vi "test1_korras.vi"() -> ()   [LabVIEW 2012]
panel:
  out "XY Graph 2":cluster{timestamp[], dbl[]}(graph)
  out "XY Graph":cluster{timestamp[], dbl[]}(graph)
  in  "Path":path
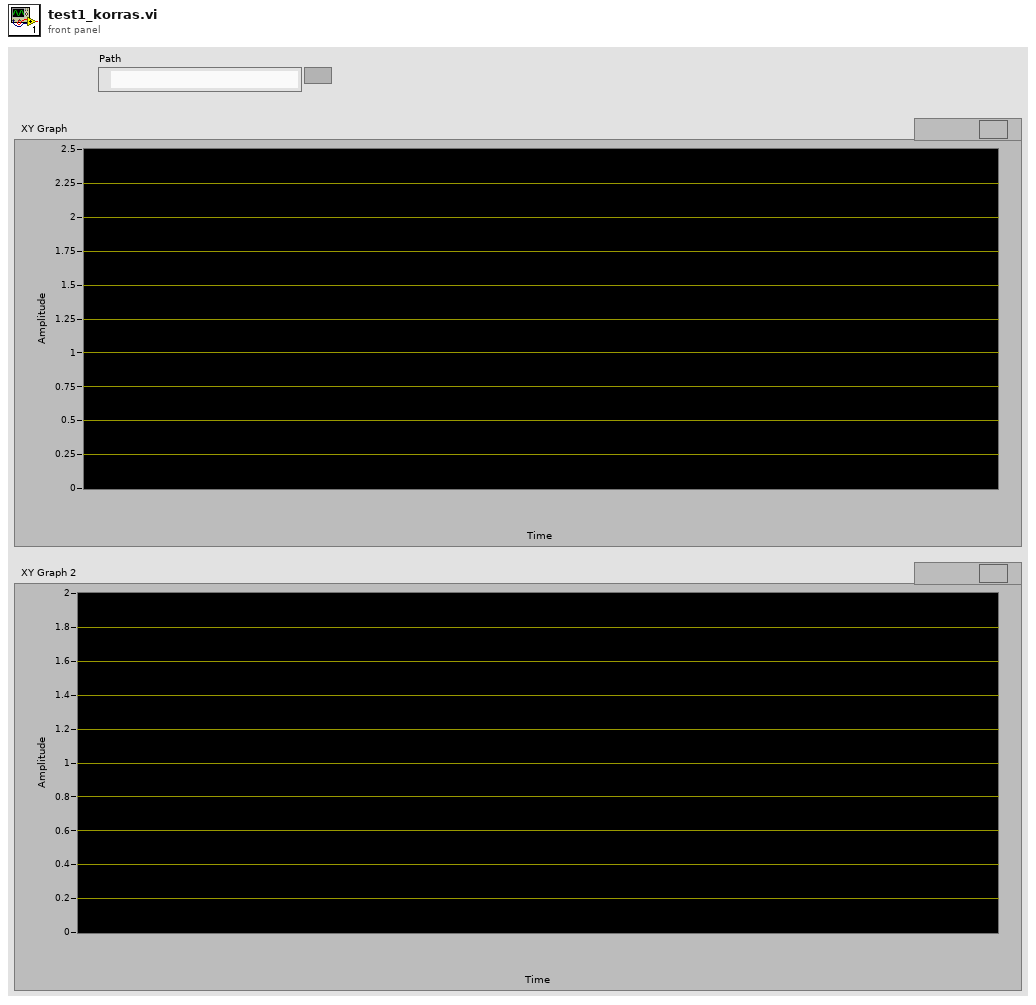
[diagram p1: front panel]
types:
  T1 = enum16{"open", "replace", "create", "open or create", "replace or create", "replace or create with confirmation"}
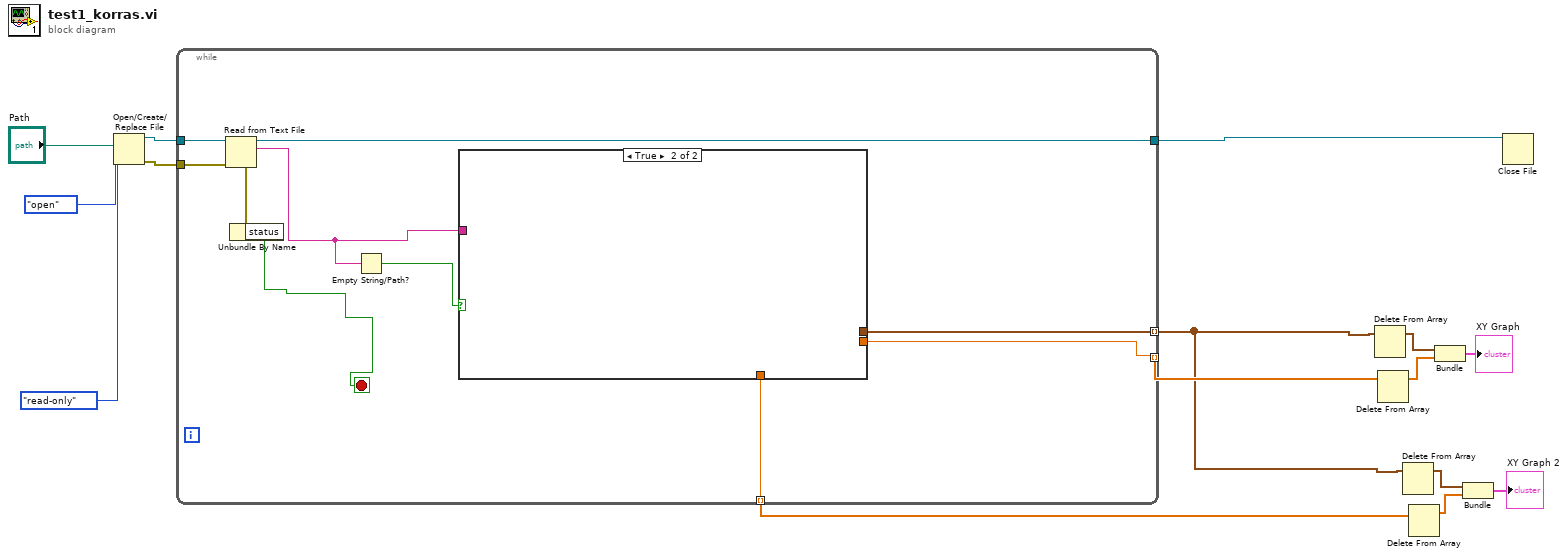
[diagram p0: block diagram]
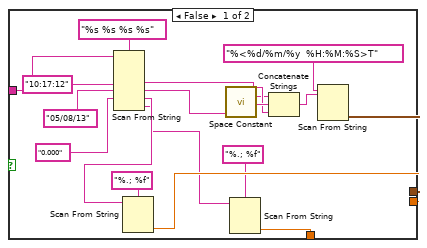
[diagram p2: hidden frame]
diagram:
  n1 = Open/Create/Replace File(file path (use dialog)="Path", operation (0:open)=T1."open", access (0:read/write)=enum16{"read/write", "read-only", "write-only"}."read-only") -> (refnum out=w14:refnum<file>, error out=w15:errorcluster)  [unwired: 3 in, 1 out]
  n2 = while {
    tunnel: w15 -> [w25]
    tunnel: w14 -> [w23]
    tunnel: [w22] -> w10
    tunnel: [w20] -> w8 mode=indexing
    tunnel: [w21] -> w1 mode=indexing
    tunnel: [w16] -> w2 mode=indexing
    stop <- w17 stop-if-true
    n3 = Read from Text File(file (use dialog)=w23, error in=w25) -> (refnum out=w22:refnum<file>, text=w19:string, error out=w24:errorcluster)  [unwired: 2 in, 1 out]
    n4 = Unbundle By Name(w24) -> ("status"=w17:bool)
    n5 = Empty String/Path?(string/path=w19) -> (empty?=w18:bool)
    n6 = case shown="True" w18 {
      tunnel: [w30 _] -> w21
      tunnel: [w29 _] -> w20
      tunnel: w19 -> [w31 _]
      tunnel: [w26 _] -> w16
      frame False {
        n7 = Scan From String(format string="%s %s %s %s", input string=w31, default 1="10:17:12", default 2="05/08/13", default 3="0.000") -> (output 1=w38:string, output 2=w37:string, output 3=w40:string, output 4=w27:string)  [unwired: 3 in, 3 out]
        n8 = Scan From String(format string="%.; %f", input string=w40) -> (output 1=w29:dbl)  [unwired: 3 in, 3 out]
        n9 = call <vilib>:"Space Constant.vi"() -> ("String"=w39:string)
        n10 = Scan From String(format string="%.; %f", input string=w27) -> (output 1=w26:dbl)  [unwired: 3 in, 3 out]
        n11 = Concatenate Strings(w37, w39, w38) -> (w35:string)
        n12 = Scan From String "Scan From String"(format string="%<%d/%m/%y  %H:%M:%S>T", input string=w35) -> (output 1=w30:timestamp)  [unwired: 3 in, 3 out]
      }
      frame True {
      }
    }
  }
  n13 = Delete From Array(array=w1) -> (array with subset deleted=w6:timestamp[])  [unwired: 2 in, 1 out]
  n14 = Delete From Array(array=w8) -> (array with subset deleted=w7:dbl[])  [unwired: 2 in, 1 out]
  n15 = Delete From Array(array=w1) -> (array with subset deleted=w3:timestamp[])  [unwired: 2 in, 1 out]
  n16 = Delete From Array(array=w2) -> (array with subset deleted=w4:dbl[])  [unwired: 2 in, 1 out]
  n17 = Bundle(w6, w7) -> (→"XY Graph":cluster{timestamp[], dbl[]})  [unwired: 1 in]
  n18 = Bundle(w3, w4) -> (→"XY Graph 2":cluster{timestamp[], dbl[]})  [unwired: 1 in]
  n19 = Close File(refnum=w10) -> ()  [unwired: 1 in, 2 out]
